vi "Read value as String.vi"(8 "error in (no error)":errorcluster, 9 "default value":string, 11 "JSON String in":refnum<class "JSON Value.lvclass">) -> (0 "error out":errorcluster, 2 "value":string)   [LabVIEW 2016, in "JSON Value.lvclass"]
doc: "Returns the value of a JSON String"
uses:
  JSON Value.lvclass
  JSON Value.lvclass/JSON Value.ctl
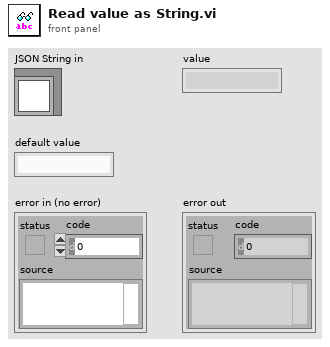
[diagram p1: front panel]
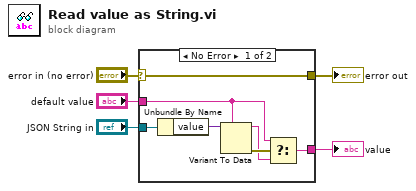
[diagram p0: block diagram]
diagram:
  n1 = case shown="No Error" "error in (no error)" {
    selector: "error in (no error)" -> [w12 w14]
    tunnel: [w12 w14] -> w4
    tunnel: "JSON String in" -> [w11 _]
    tunnel: [w6 w13] -> w2
    tunnel: "default value" -> [w8 w13]
    frame No Error {
      n2 = Unbundle By Name(w11) -> ("value"=w10:variant)
      n3 = Variant To Data(type=w8, Variant=w10) -> (data=w7:string, error out=w9:errorcluster)  [unwired: 1 in]
      n4 = Select(t=w8, s=w9, f=w7) -> (s? t:f=w6:string)
    }
    frame Error {
    }
  }
  "error out" <- w4
  "value" <- w2
